vi "FPGA.vi"() -> ()   [LabVIEW 2015]
uses:
  SPI v2/ADXL345 Output.ctl
  <userlib>/_NI SPI IP/FPGA/Controllers/Public/Transfer Settings.ctl
  SPI v2/ADXL345 SPI Statechart.lvsc/Outputs.ctl
  <vilib>/Platform/TimedLoop/XDataNode/timing_clust.ctl
  <vilib>/Platform/TimedLoop/XDataNode/nitl_modes.ctl
  <vilib>/Platform/TimedLoop/XDataNode/wakeup.ctl
  <userlib>/_NI SPI IP/FPGA/Controllers/Public/Spi Master Inputs.ctl
  SPI v2/ADXL345 SPI Statechart.lvsc/Inputs.ctl
  <vilib>/rvi/Emulation/niFpgaGetClockAttributes.vi
  <vilib>/rvi/Emulation/niFpgaSctlEmulationGetInTimedLoop.vi
  <vilib>/rvi/Emulation/niFpgaEmulationReportErrorSimple.vi
  <vilib>/rvi/eio/common/nirviEmuTemplateMethod_errors.vi
  FPGA Globals.vi
  <vilib>/rvi/Emulation/niFpgaCriticalErrorInLSC.vi
  <vilib>/rvi/Emulation/niFpgaProcessEmulError.vi
  SPI v2/ADXL345 SPI Statechart.lvsc/CompanionDiagram.vi/7/SC Main.vi
  <vilib>/eio/EIONode/EIONode.xnode
  <vilib>/rvi/Analysis/measure/butterworth/XNode/niFpgaButterworthFilter.xnode
  <vilib>/Platform/TimedLoop/XDataNode/XDataNode.xnode
  SPI v2/ADXL345 SPI Statechart.lvsc/Trigger.ctl
  <vilib>/Statechart/Infrastructure/RTStatechart/RunTime SCN.xnode
  SPI v2/ADXL345 SPI Statechart.lvsc
  <vilib>/Platform/TimedLoop/XDataNode/XDNodeRunTimeDep.lvlib
  <userlib>/_NI SPI IP/FPGA/Controllers/NI SPI IP FPGA.lvlib
panel:
  out "PWM Out OFF":bool=TRUE
  out "PWM Duty":fxp<+/-,23,14>=336.0
  out "PWM Loop Clock":fxp<+,16,16>
  out "PWM Out ON":bool=TRUE
  in  "BMSTemp":fxp<+,16,8>
  in  "bSBRIOOK3":bool
  in  "bPO2":bool
  in  "bPO3":bool
  out "VHighCurrent":fxp<+/-,36,9>
  out "VLowCurrent":fxp<+/-,36,9>
  in  "bDCDCDisable":bool
  in  "bLapBeaconPickupEnable":bool
  in  "bWheelSpeedsEnable":bool
  out "bLapBeaconPickup":bool
  out "tLapDelta":u32
  in  "bResetFastestLap":bool
  out "tFastestLap":u32
  in  "tLapReference":u32
  in  "bWheelFRFail":bool
  in  "bWheelFLFail":bool
  out "ADXL345 Output":T1
  out "rSlipFR":fxp<+/-,12,1>
  out "rSlipFL":fxp<+/-,12,1>
  out "rSlipRR":fxp<+/-,12,1>
  out "rSlipRL":fxp<+/-,12,1>
  out "sLap":fxp<+,32,12>
  out "vCar":fxp<+/-,33,19>
  out "vAxleF":fxp<+/-,33,19>
  in  "bAccel":bool
  out "vWheelHighest":fxp<+/-,32,18>
  out "vWheelLowest":fxp<+/-,32,18>
  out "vWheelFL":fxp<+/-,32,18>
  out "vWheelFR":fxp<+/-,32,18>
  out "vWheelRL":fxp<+/-,32,18>
  out "vWheelRR":fxp<+/-,32,18>
  in  "Tire Diameter(m)":fxp<+,16,1>
  out "nWheelRR":fxp<+/-,29,16>
  out "nWheelRL":fxp<+/-,29,16>
  out "nWheelFR":fxp<+/-,29,16>
  out "nWheelFL":fxp<+/-,29,16>
  out "NLap":u8
  in  "bResetNLap":bool
  out "aSteerWheel":fxp<+/-,22,10>=124.904541015625
  in  "VSteerWheelMiddle":fxp<+/-,26,5>=0.34827280044555664
  out "bBrakeFOK":bool
  out "bBrakeROK":bool
  out "bLowCurrentOK":bool
  out "bHighCurrentOK":bool
  out "pBrakeF":fxp<+,26,13>
  out "pBrakeR":fxp<+,26,13>
  out "ILowCurrent":fxp<+/-,19,15>=4.375
  out "IHighCurrent":fxp<+/-,19,15>=-20.75
  out "VShockFL":fxp<+/-,24,5>=0.3892974853515625
  out "VShockFR":fxp<+/-,24,5>=0.3425788879394531
  out "VShockRL":fxp<+/-,24,5>=0.3444976806640625
  out "VShockRR":fxp<+/-,24,5>=0.3793773651123047
  in  "bBrakeLight":bool=TRUE
  out "tWheelFLPeriod":u32
  out "tWheelFRPeriod":u32
  out "tWheelRRPeriod":u32
  out "tWheelRLPeriod":u32
  out "bWheelFLStopped":bool=TRUE
  out "bWheelFRStopped":bool=TRUE
  out "bWheelRLStopped":bool=TRUE
  out "bWheelRRStopped":bool=TRUE
  out "VBrakePressureF":fxp<+/-,24,5>=0.4808177947998047
  out "VBrakePressureR":fxp<+/-,24,5>=0.4820976257324219
  out "bWheelFL":bool
  out "bWheelFR":bool
  out "bWheelRR":bool
  out "bWheelRL":bool
  out "V5VSupply":fxp<+/-,24,5>
  in  "tLapMin":u32=15000
  out "tLastLap":u32
  out "bNewLap":bool
  out "tCurrentLap":u32
  in  "bMotorControllerEnable":bool
  out "bTSMSOutStatus":bool
  in  "bSBRIOOK1":bool
  in  "bSBRIOOK2":bool
  out "bBSPDOK":bool
  out "bIMDOK":bool
  out "bBMSOK":bool
  in  "bPosAIREnable":bool
  out "bTSMSInStatus":bool
  in  "bRTDSEnable":bool
  in  "bCoolantPumpEnable":bool
  in  "rTPS1Min":fxp<+,16,4>=0.39990234375
  in  "rTPS1Max":fxp<+,16,4>=0.6201171875
  in  "rTPS2Min":fxp<+,16,4>=0.489990234375
  in  "rTPS2Max":fxp<+,16,4>=0.27001953125
  out "rTPS1":fxp<+/-,31,22>
  out "VTPS1":fxp<+/-,36,9>=3.619058609008789
  out "rTPS2":fxp<+/-,31,22>
  out "VTPS2":fxp<+/-,36,9>=1.0001773834228516
  out "rThrottle":fxp<+/-,33,22>
  out "bTPSInRange":bool
  out "bTPSConsistent":bool
  out "rTPS1Unscaled":fxp<+/-,16,1>
  out "rTPS2Unscaled":fxp<+/-,16,1>
  out "TSBRIO":fxp<+,19,8>=27.25 format="%.10g"
  out "bFPGALED":bool
  out "VsbRIOSupply":fxp<+/-,25,6>=13.101043701171875
  in  "VSupplyOffset":fxp<+,12,4>=8.890625
  in  "stop":bool
  out "Tick Count(mSec)":u32
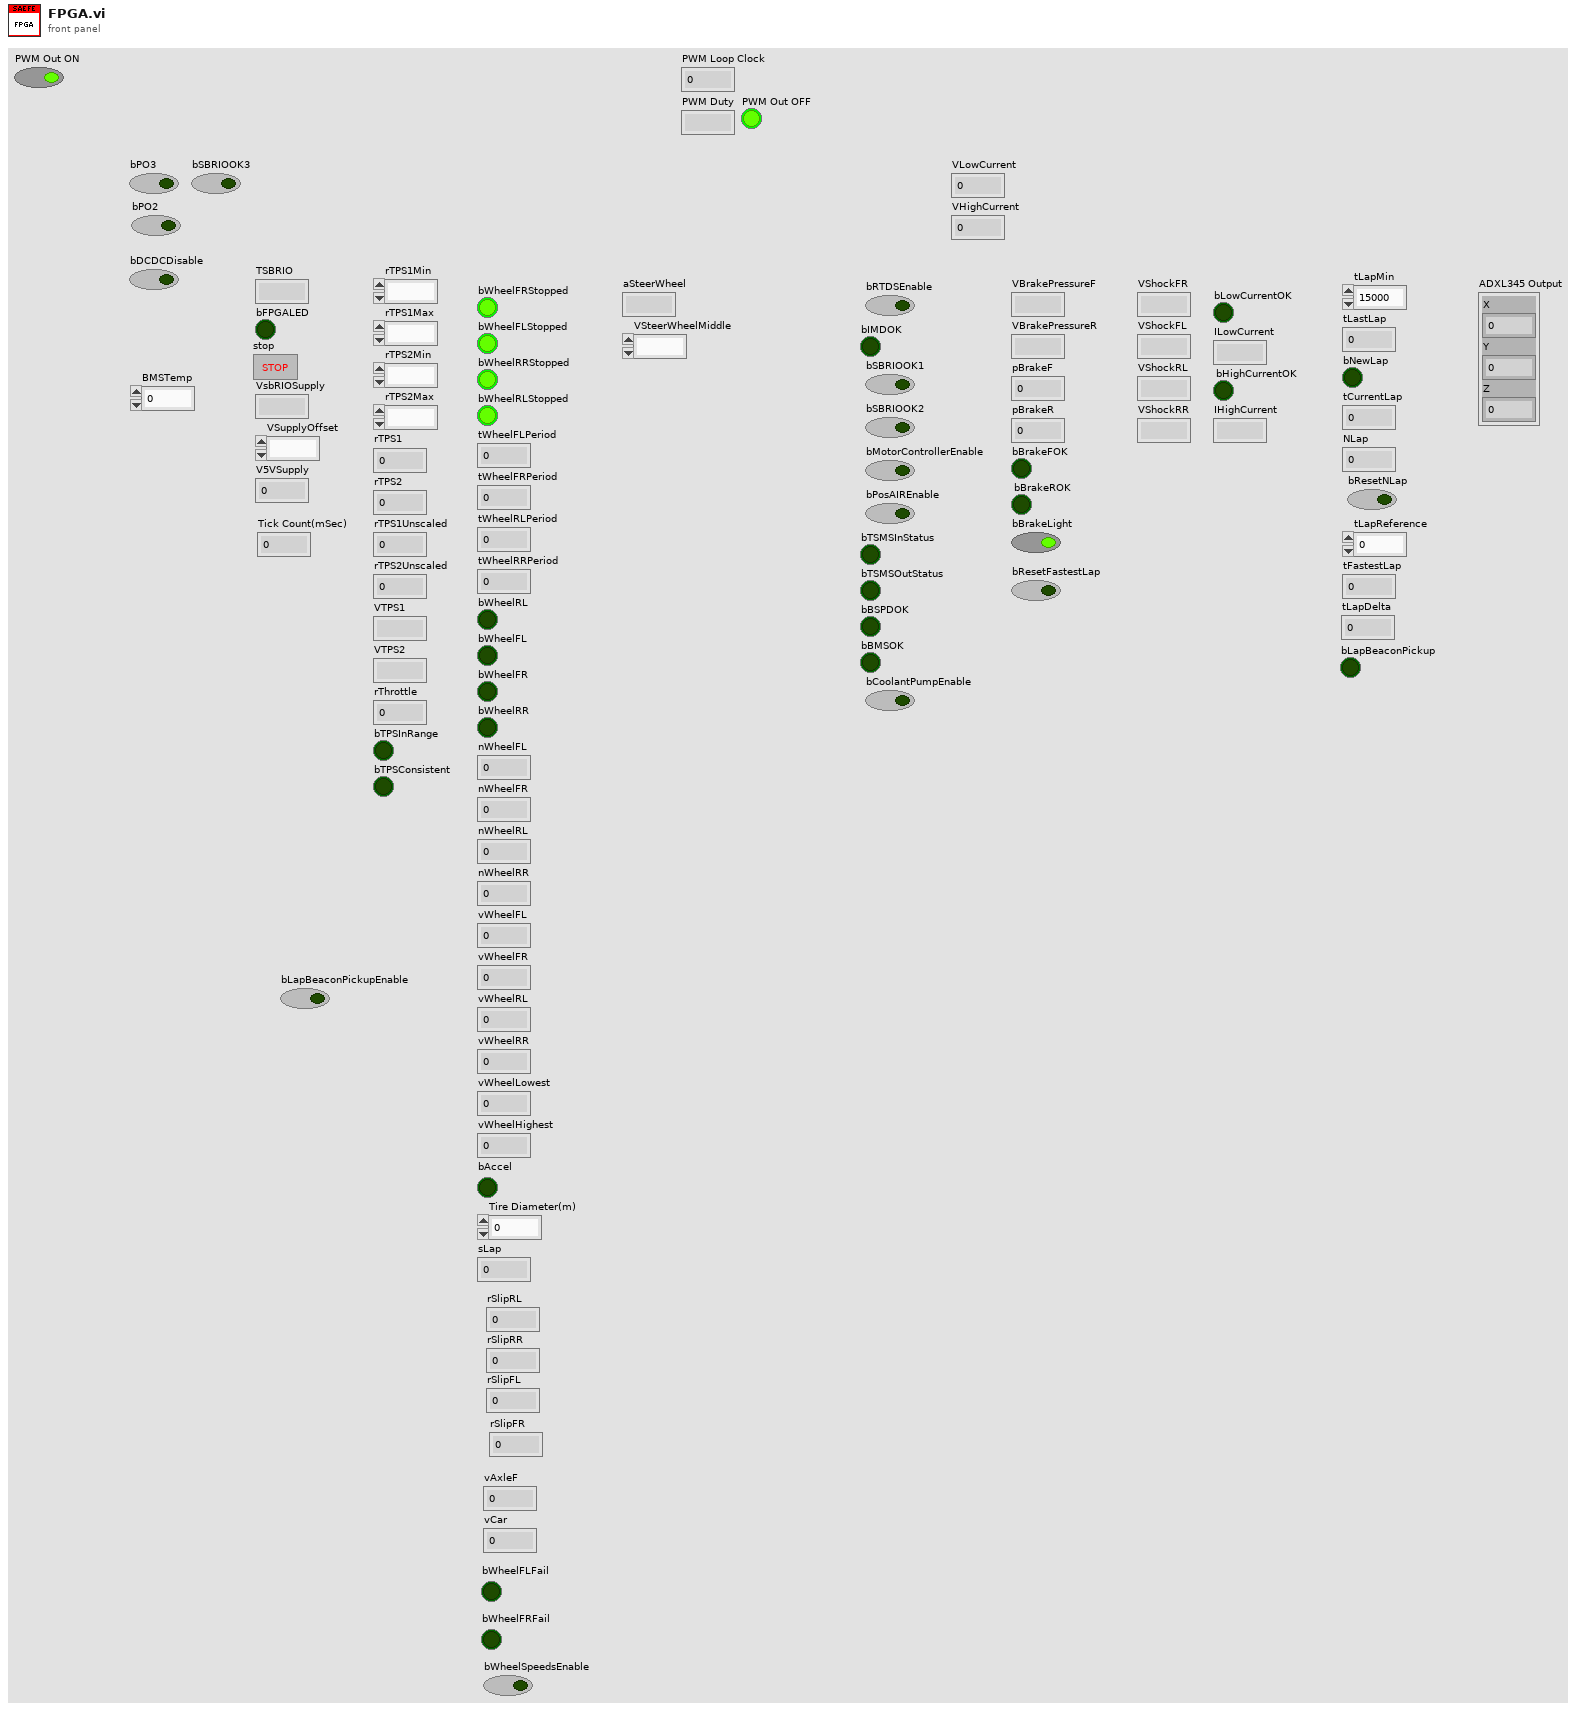
[diagram p1: front panel]
types:
  T1 = typedef "ADXL345 Output.ctl" = cluster{"X":fxp<+/-,14,4>, "Y":fxp<+/-,14,4>, "Z":fxp<+/-,14,4>}
  T2 = typedef "ADXL345 SPI Statechart.lvsc/Outputs.ctl" = cluster{"Transfer Length (bits)":u8, "start strobe":bool, "data to write":u64, "ADXL345 Output":T1}
  T3 = typedef "NI SPI IP FPGA.lvlib/Transfer Settings.ctl" = cluster{"Divide Value":u8, "Transfer Length (bits)":u8, "CS Asserted Polarity":bool, "Clock Polarity (CPOL)":bool, "Clock Phase (CPHA)":bool, "Lengthen MISO Setup":bool, "Direction Change Bit":u8, "MOSI Starts as Output":bool, "Tristatable MOSI":bool}
  T4 = typedef "ADXL345 SPI Statechart.lvsc/Inputs.ctl" = cluster{"read data valid":bool, "read data":u64, "ready for input":bool}
  T5 = typedef "NI SPI IP FPGA.lvlib/Spi Master Inputs.ctl" = cluster{"MISO":bool}
  T6 = typedef "XDNodeRunTimeDep.lvlib/timing_clust.ctl" = cluster{"Expected End [f-1]":u64, "Actual End [f-1]":u64, "Finished Late? [f-1]":bool, "Expected End [i-1]":u64, "Actual End [i-1]":u64, "Finished Late? [i-1]":bool, "Expected Start [i]":u64, "Actual Start [i]":u64, "Expected Start [f]":u64, "Actual Start [f]":u64, "Source Name":string, "Structure Name":string, "Period":i64, "Deadline":i64, "Offset":i64, "Start":i64, "Priority":i32, "Timeout":i32, "Mode":T7, "Wakeup Reason":T8, "Error":errorcluster, "Source Type":string, "Secondary Source Type":string, "Global End Time":u64, "Global Start Time":u64, "Frame Duration":u64, "Iteration Duration":u64, "Assigned CPU":i32, "I/O Scan Engine Mode":u32}
  T7 = typedef "XDNodeRunTimeDep.lvlib/nitl_modes.ctl" = enum32{"No Change", "Process missed periods, maintain original phase", "Discard missed periods, maintain original phase", "Process missed periods, ignore original phase", "Discard missed periods, ignore original phase"}
  T8 = typedef "XDNodeRunTimeDep.lvlib/wakeup.ctl" = enum32{"Normal", "Aborted", "Asynchronous wakeup", "Timing source error", "Timed loop error", "Timeout"}
  T9 = typedef "NI SPI IP FPGA.lvlib/Spi Master Outputs.ctl" = cluster{"Chip Select":bool, "Clock":bool, "MOSI":bool, "MOSI OE":bool}
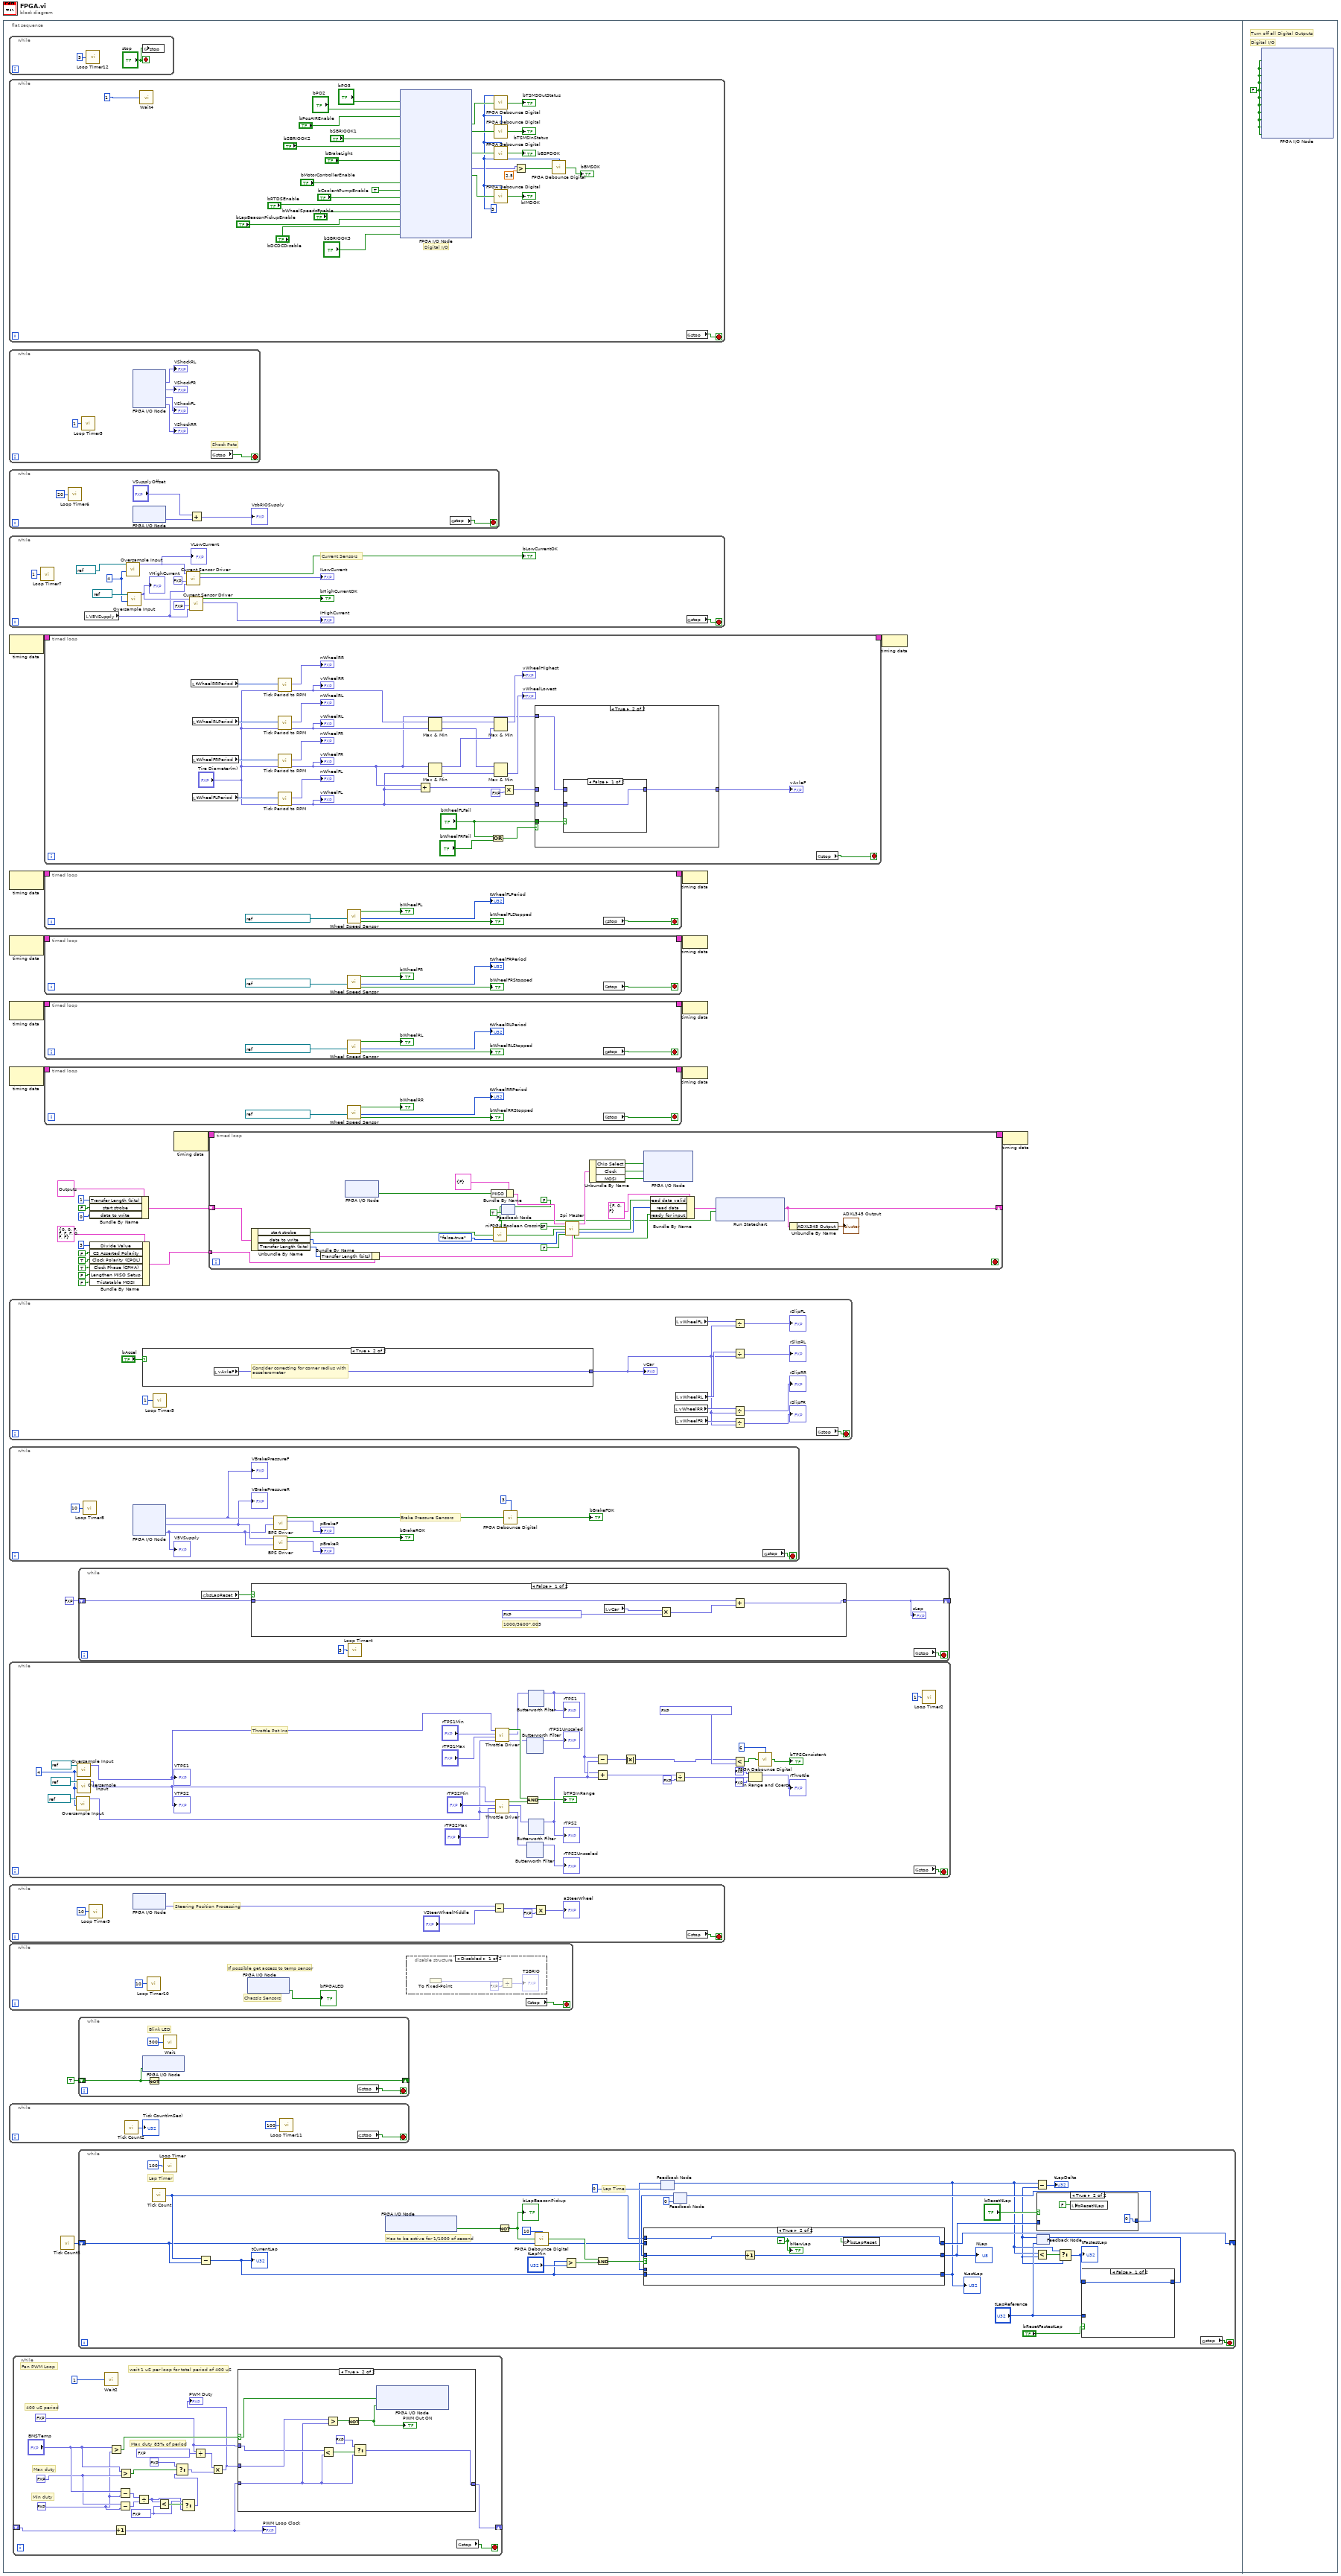
[diagram p0: block diagram]
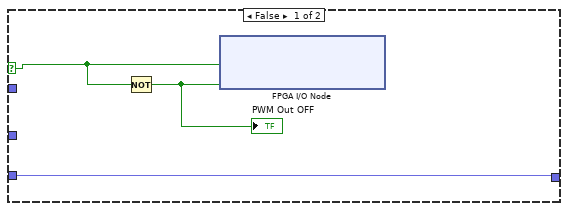
[diagram p2: hidden frame]
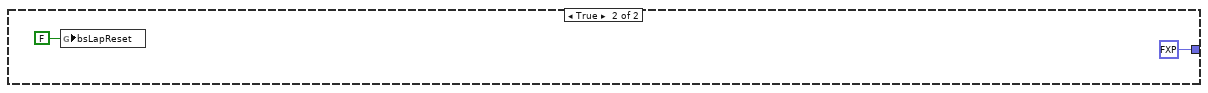
[diagram p3: hidden frame]
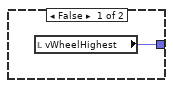
[diagram p4: hidden frame]
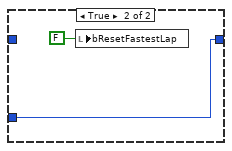
[diagram p7: hidden frame]
diagram:
  n1 = flat-sequence {
    frame #0 {
      n2 = while {
        stop <- "stop" stop-if-true
        n3 = call "Loop Timer12"("Count(mSec)"=u32 5) -> ()  [unwired: 1 out]
        n4 = global write "FPGA Globals.vi" "stop"("stop") -> ()
      }
      n5 = while {
        stop <- w387 stop-if-true
        w364 = u16 3 ("Cycles to Filter")
        # "Digital I/O"
        n6 = call "Wait4"("Count(mSec)"=u32 1) -> ()  [unwired: 1 out]
        n7 = xnode "FPGA I/O Node"("RMC Connector/DIO40"="bPO3", "RMC Connector/DIO42"="bPO2", "RMC Connector/DIO8"="bPosAIREnable", "RMC Connector/DIO5"="bSBRIOOK1", "RMC Connector/DIO6"="bSBRIOOK2", "RMC Connector/DIO11"="bBrakeLight", "RMC Connector/DIO33"="bMotorControllerEnable", "RMC Connector/DIO14"=TRUE, "RMC Connector/DIO41"="bCoolantPumpEnable", "RMC Connector/DIO43"="bRTDSEnable", "RMC Connector/DIO83"="bWheelSpeedsEnable", "RMC Connector/DIO4"="bLapBeaconPickupEnable", "RMC Connector/DIO45"="bDCDCDisable", "RMC Connector/DIO37"="bSBRIOOK3") -> ("RMC Connector/DIO7"=w385:bool, "RMC Connector/DIO39"=w383:bool, "RMC Connector/DIO1"=w372:bool, "AI8"=w362:fxp<+/-,24,5>, "RMC Connector/DIO95"=w379:bool)  [unwired: 19 in, 19 out]
        n8 = call "FPGA Debounce Digital.vi"("Input Signal"=w385, "Cycles to Filter"=w364) -> ("Output Filtered Signal"=→"bTSMSOutStatus":bool)
        n9 = call "FPGA Debounce Digital.vi"("Input Signal"=w383, "Cycles to Filter"=w364) -> ("Output Filtered Signal"=→"bTSMSInStatus":bool)
        n10 = call "FPGA Debounce Digital.vi"("Input Signal"=w372, "Cycles to Filter"=w364) -> ("Output Filtered Signal"=→"bBSPDOK":bool)
        n11 = call "FPGA Debounce Digital.vi"("Input Signal"=w379, "Cycles to Filter"=w364) -> ("Output Filtered Signal"=→"bIMDOK":bool)
        n12 = Greater?(x=w362, y=sgl 2.5) -> (0:w361:bool)
        n13 = call "FPGA Debounce Digital.vi"("Input Signal"=w361, "Cycles to Filter"=w364) -> ("Output Filtered Signal"=→"bBMSOK":bool)
        n14 = global read "FPGA Globals.vi" "stop"() -> (w387:bool)
      }
      n15 = while {
        stop <- w262 stop-if-true
        # "Shock Pots"
        n16 = call "Loop Timer5"("Count(mSec)"=u32 1) -> ()  [unwired: 1 out]
        n17 = xnode "FPGA I/O Node"() -> ("AI9"=→"VShockRL":fxp<+/-,24,5>, "AI10"=→"VShockFR":fxp<+/-,24,5>, "AI11"=→"VShockFL":fxp<+/-,24,5>, "AI8"=→"VShockRR":fxp<+/-,24,5>)  [unwired: 4 in, 4 out]
        n18 = global read "FPGA Globals.vi" "stop"() -> (w262:bool)
      }
      n19 = while {
        stop <- w247 stop-if-true
        n20 = call "Loop Timer6"("Count(mSec)"=u32 20) -> ()  [unwired: 1 out]
        n21 = xnode "FPGA I/O Node"() -> ("AI0"=w250:fxp<+/-,24,5>)  [unwired: 1 in, 1 out]
        n22 = Add(x="VSupplyOffset", y=w250) -> (x+y=→"VsbRIOSupply":fxp<+/-,25,6>)
        n23 = global read "FPGA Globals.vi" "stop"() -> (w247:bool)
      }
      n24 = while {
        stop <- w274 stop-if-true
        w271 = u8 4 ("NSamples")
        # "Current Sensors"
        n25 = call "Loop Timer7"("Count(mSec)"=u32 1) -> ()  [unwired: 1 out]
        n26 = local read "V5VSupply"() -> (w269:fxp<+/-,24,5>)
        n27 = call "Oversample Input.vi"("NSamples"=w271, "Channel"=refnum<k21> "AI2" ("FPGA I/O In")) -> ("Output"=w267:fxp<+/-,36,9>)  [unwired: 9 in]
        "VLowCurrent" <- w267
        n28 = call "Oversample Input.vi"("NSamples"=w271, "Channel"=refnum<k21> "AI1") -> ("Output"=w270:fxp<+/-,36,9>)  [unwired: 9 in]
        "VHighCurrent" <- w270
        n29 = call "Current Sensor Driver.vi"("VSupply"=w269, "IRange"=fxp<+,27,10> 50.0 ("Range"), "VInput"=w267) -> ("ISensor"=→"ILowCurrent":fxp<+/-,19,15>, "bSensorOK"=→"bLowCurrentOK":bool)  [unwired: 7 in]
        n30 = call "Current Sensor Driver.vi"("VSupply"=w269, "IRange"=fxp<+,27,10> 600.0 ("Range"), "VInput"=w270) -> ("ISensor"=→"IHighCurrent":fxp<+/-,19,15>, "bSensorOK"=→"bHighCurrentOK":bool)  [unwired: 7 in]
        n31 = global read "FPGA Globals.vi" "stop"() -> (w274:bool)
      }
      n32 = node-c288() -> (w18:T6)  [unwired: 1 in]
      n33 = node-c288() -> (w27:T6)  [unwired: 1 in]
      n34 = node-c288() -> (w25:T6)  [unwired: 1 in]
      n35 = node-c288() -> (w23:T6)  [unwired: 1 in]
      n36 = node-c288() -> (w21:T6)  [unwired: 1 in]
      n37 = while {
        stop <- w122 stop-if-true
        n38 = case shown="True" "bAccel" {
          tunnel: [w123 w124] -> w112
          frame False {
            n39 = local read "vWheelHighest"() -> (w123:fxp<+/-,32,18>)
          }
          frame True {
            # "Consider correcting for corner radius with\naccelerometer"
            n40 = local read "vAxleF"() -> (w124:fxp<+/-,33,19>)
          }
        }
        "vCar" <- w112
        n41 = call "Loop Timer3"("Count(mSec)"=u32 1) -> ()  [unwired: 1 out]
        n42 = local read "vWheelRR"() -> (w117:fxp<+/-,32,18>)
        n43 = local read "vWheelFL"() -> (w115:fxp<+/-,32,18>)
        n44 = local read "vWheelRL"() -> (w119:fxp<+/-,32,18>)
        n45 = local read "vWheelFR"() -> (w113:fxp<+/-,32,18>)
        n46 = Divide(x=w115, y=w112) -> (x/y=→"rSlipFL":fxp<+/-,12,1>)
        n47 = Divide(x=w119, y=w112) -> (x/y=→"rSlipRL":fxp<+/-,12,1>)
        n48 = Divide(x=w117, y=w112) -> (x/y=→"rSlipRR":fxp<+/-,12,1>)
        n49 = Divide(x=w113, y=w112) -> (x/y=→"rSlipFR":fxp<+/-,12,1>)
        n50 = global read "FPGA Globals.vi" "stop"() -> (w122:bool)
      }
      n51 = while {
        stop <- w286 stop-if-true
        # "Brake Pressure Sensors"
        n52 = call "Loop Timer8"("Count(mSec)"=u32 10) -> ()  [unwired: 1 out]
        n53 = xnode "FPGA I/O Node"() -> ("AI3"=w291:fxp<+/-,24,5>, "AI4"=w289:fxp<+/-,24,5>, "AI12"=w284:fxp<+/-,24,5>)  [unwired: 3 in, 3 out]
        "VBrakePressureF" <- w291
        "VBrakePressureR" <- w289
        "V5VSupply" <- w284
        n54 = call "BPS Driver.vi"("Supply Voltage"=w284, "Signal In"=w291) -> ("Brake Pressure (psi)"=→"pBrakeF":fxp<+,26,13>, "Sensor OK?"=w283:bool)  [unwired: 8 in]
        n55 = call "BPS Driver.vi"("Supply Voltage"=w284, "Signal In"=w289) -> ("Brake Pressure (psi)"=→"pBrakeR":fxp<+,26,13>, "Sensor OK?"=→"bBrakeROK":bool)  [unwired: 8 in]
        n56 = call "FPGA Debounce Digital.vi"("Input Signal"=w283, "Cycles to Filter"=u16 3) -> ("Output Filtered Signal"=→"bBrakeFOK":bool)
        n57 = global read "FPGA Globals.vi" "stop"() -> (w286:bool)
      }
      n58 = while {
        stop <- w318 stop-if-true
        w300 = u8 4 ("NSamples")
        # "Throttle Pot Ins"
        n59 = call "Oversample Input.vi"("NSamples"=w300, "Channel"=refnum<k21> "AI12") -> ("Output"=w298:fxp<+/-,36,9>)  [unwired: 9 in]
        n60 = call "Oversample Input.vi"("NSamples"=w300, "Channel"=refnum<k21> "AI6") -> ("Output"=w299:fxp<+/-,36,9>)  [unwired: 9 in]
        "VTPS2" <- w299
        n61 = call "Oversample Input.vi"("NSamples"=w300, "Channel"=refnum<k21> "AI5") -> ("Output"=w296:fxp<+/-,36,9>)  [unwired: 9 in]
        "VTPS1" <- w296
        n62 = call "Throttle Driver.vi"("Reference Voltage In"=w298, "Throttle Max"="rTPS1Max", "Throttle Min"="rTPS1Min", "Throttle Voltage In"=w296) -> ("Unscaled Throttle Percent"=w313:fxp<+/-,16,1>, "Throttle Percent"=w306:fxp<+/-,27,18>, "In Range"=w322:bool)  [unwired: 5 in]
        n63 = call "Throttle Driver.vi"("Reference Voltage In"=w298, "Throttle Max"="rTPS2Max", "Throttle Min"="rTPS2Min", "Throttle Voltage In"=w299) -> ("Unscaled Throttle Percent"=w311:fxp<+/-,16,1>, "Throttle Percent"=w309:fxp<+/-,27,18>, "In Range"=w321:bool)  [unwired: 5 in]
        n64 = xnode "Butterworth Filter"("input data"=w313) -> ("output data"=→"rTPS1Unscaled":fxp<+/-,16,1>)  [unwired: 2 in]
        n65 = xnode "Butterworth Filter"("input data"=w311) -> ("output data"=→"rTPS2Unscaled":fxp<+/-,16,1>)  [unwired: 2 in]
        n66 = Compound Arithmetic op=AND(w322, w321) -> (→"bTPSInRange":bool)
        n67 = xnode "Butterworth Filter"("input data"=w306) -> ("output data"=w305:fxp<+/-,31,22>)  [unwired: 2 in]
        "rTPS1" <- w305
        n68 = xnode "Butterworth Filter"("input data"=w309) -> ("output data"=w308:fxp<+/-,31,22>)  [unwired: 2 in]
        "rTPS2" <- w308
        n69 = Subtract(x=w305, y=w308) -> (x-y=w317:fxp<+/-,32,23>)
        n70 = Add(x=w305, y=w308) -> (x+y=w324:fxp<+/-,32,23>)
        n71 = Absolute Value(x=w317) -> (abs(x)=w293:fxp<+,31,22>)
        n72 = Divide(x=w324, y=fxp<+,1,2> 2.0) -> (x/y=w307:fxp<+/-,33,22>)
        n73 = Less?(x=w293, y=fxp<+/-,46,20> 0.09999999403953552) -> (x < y?=w295:bool)
        n74 = In Range and Coerce(upper limit=fxp<+/-,33,22> 1.0, x=w307, lower limit=fxp<+/-,33,22> 0.0) -> (coerced(x)=→"rThrottle":fxp<+/-,33,22>)  [unwired: 1 out]
        n75 = call "FPGA Debounce Digital.vi"("Input Signal"=w295, "Cycles to Filter"=i16 6) -> ("Output Filtered Signal"=→"bTPSConsistent":bool)
        n76 = global read "FPGA Globals.vi" "stop"() -> (w318:bool)
        n77 = call "Loop Timer2"("Count(mSec)"=u32 1) -> ()  [unwired: 1 out]
      }
      n78 = while {
        stop <- w390 stop-if-true
        # "Steering Position Processing"
        n79 = call "Loop Timer9"("Count(mSec)"=u32 10) -> ()  [unwired: 1 out]
        n80 = xnode "FPGA I/O Node"() -> ("AI14"=w395:fxp<+/-,24,5>)  [unwired: 1 in, 1 out]
        n81 = Subtract(x=w395, y="VSteerWheelMiddle") -> (x-y=w393:fxp<+/-,27,6>)
        n82 = Multiply(x=w393, y=fxp<+,4,7> 72.0) -> (x*y=→"aSteerWheel":fxp<+/-,22,10>)
        n83 = global read "FPGA Globals.vi" "stop"() -> (w390:bool)
      }
      n84 = while {
        stop <- w257 stop-if-true
        # "If possible get access to temp sensor"
        # "Chassis Sensors"
        n85 = call "Loop Timer10"("Count(mSec)"=u32 10) -> ()  [unwired: 1 out]
        n86 = xnode "FPGA I/O Node"() -> ("FPGA LED"=→"bFPGALED":bool)  [unwired: 1 in, 1 out]
        n87 = disable-structure shown="Disabled" {
          frame Disabled {
            n88 = To Fixed-Point() -> (fixed-point=w259:fxp<+/-,16,9>)  [unwired: 2 in]
            n89 = Divide(x=w259, y=fxp<+/-,16,9> 4.0) -> (x/y=→"TSBRIO":fxp<+,19,8>)
          }
          frame Enabled {
          }
        }
        n90 = global read "FPGA Globals.vi" "stop"() -> (w257:bool)
      }
      n91 = while {
        stop <- w242 stop-if-true
        n92 = call "Tick Count2"() -> ("Tick Count(mSec)"=→"Tick Count(mSec)":u32)
        n93 = call "Loop Timer11"("Count(uSec)"=u32 100) -> ()  [unwired: 1 out]
        n94 = global read "FPGA Globals.vi" "stop"() -> (w242:bool)
      }
      n95 = while {
        shift-right: [w41] -> _
        shift-left: _ -> [w42]
        stop <- w40 stop-if-true
        w31 = fxp<+,5,-1> 0.40625
        w38 = fxp<+,5,9> 400.0
        w47 = fxp<+,3,6> 40.0 ("Temp 2")
        w48 = fxp<+,6,6> 55.0 ("Temp 2")
        # "400 uS period"
        # "wait 1 uS per loop for total period of 400 uS"
        # "Max duty 85% of period"
        # "Fan PWM Loop"
        # "Min duty"
        # "Max duty"
        n96 = call "Wait2"("Count(uSec)"=u8 1) -> ()  [unwired: 1 out]
        n97 = Greater?(x="BMSTemp", y=w47) -> (0:w43:bool)
        n98 = Increment(x=w42) -> (x+1=w36:fxp<+,16,16>)
        "PWM Loop Clock" <- w36
        n99 = Subtract(x="BMSTemp", y=w47) -> (x-y=w34:fxp<+/-,17,9>)
        n100 = Subtract(x=w48, y=w47) -> (x-y=w33:fxp<+,4,4>)
        n101 = Greater?(x="BMSTemp", y=w48) -> (0:w50:bool)
        n102 = Divide(x=w34, y=w33) -> (x/y=w30:fxp<+/-,17,5>)
        n103 = Less?(x=w30, y=w31) -> (x < y?=w32:bool)
        n104 = Select(t=w31, s=w32, f=w30) -> (s? t:f=w29:fxp<+/-,17,5>)
        n105 = Select(t=fxp<+,1,1> 1.0, s=w50, f=w29) -> (s? t:f=w46:fxp<+/-,17,5>)
        n106 = Divide(x=w38, y=fxp<+,19,1> 1.1764717102050781 ("Temp 2")) -> (x/y=w44:fxp<+,6,9>)
        n107 = Multiply(x=w44, y=w46) -> (x*y=w35:fxp<+/-,23,14>)
        "PWM Duty" <- w35
        n108 = case shown="True" w43 {
          selector: w43 -> [w52 w62]
          tunnel: w35 -> [_ w61]
          tunnel: w36 -> [w53 w56]
          tunnel: [w53 w58] -> w41
          tunnel: w38 -> [_ w57]
          frame False {
            n109 = Not(x=w52) -> (.not. x?=w51:bool)
            "PWM Out OFF" <- w51
            n110 = xnode "FPGA I/O Node"("RMC Connector/DIO9"=w52, "RMC Connector/DIO10"=w51) -> ()  [unwired: 2 in, 2 out]
          }
          frame True {
            n111 = Less?(x=w57, y=w56) -> (x < y?=w59:bool)
            n112 = Greater?(x=w61, y=w56) -> (0:w55:bool)
            n113 = Not(x=w55) -> (.not. x?=w54:bool)
            "PWM Out ON" <- w54
            n114 = Select(t=fxp<+,1,1> 0.0, s=w59, f=w56) -> (s? t:f=w58:fxp<+,16,16>)
            n115 = xnode "FPGA I/O Node"("RMC Connector/DIO9"=w62, "RMC Connector/DIO10"=w54) -> ()  [unwired: 2 in, 2 out]
          }
        }
        n116 = global read "FPGA Globals.vi" "stop"() -> (w40:bool)
      }
      n117 = timed-loop {
        timing: w18 -> [_]
        timing-out: [_] -> w17
        stop <- w145 stop-if-true
        n118 = local read "tWheelRRPeriod"() -> (w146:u32)
        n119 = local read "tWheelRLPeriod"() -> (w147:u32)
        n120 = local read "tWheelFRPeriod"() -> (w148:u32)
        n121 = local read "tWheelFLPeriod"() -> (w149:u32)
        n122 = call "Tick Period to RPM.vi"("Tire Diameter(m)"="Tire Diameter(m)", "Tick Period"=w146) -> ("vWheel"=w142:fxp<+/-,32,18>, "nWheel"=→"nWheelRR":fxp<+/-,29,16>)  [unwired: 8 in]
        "vWheelRR" <- w142
        n123 = call "Tick Period to RPM.vi"("Tire Diameter(m)"="Tire Diameter(m)", "Tick Period"=w147) -> ("vWheel"=w141:fxp<+/-,32,18>, "nWheel"=→"nWheelRL":fxp<+/-,29,16>)  [unwired: 8 in]
        "vWheelRL" <- w141
        n124 = call "Tick Period to RPM.vi"("Tire Diameter(m)"="Tire Diameter(m)", "Tick Period"=w148) -> ("vWheel"=w128:fxp<+/-,32,18>, "nWheel"=→"nWheelFR":fxp<+/-,29,16>)  [unwired: 8 in]
        "vWheelFR" <- w128
        n125 = call "Tick Period to RPM.vi"("Tire Diameter(m)"="Tire Diameter(m)", "Tick Period"=w149) -> ("vWheel"=w127:fxp<+/-,32,18>, "nWheel"=→"nWheelFL":fxp<+/-,29,16>)  [unwired: 8 in]
        "vWheelFL" <- w127
        n126 = Add(x=w128, y=w127) -> (x+y=w134:fxp<+/-,33,19>)
        n127 = Max & Min(x=w142, y=w141) -> (max(x,y)=w139:fxp<+/-,32,18>, min(x,y)=w138:fxp<+/-,32,18>)
        n128 = Max & Min(x=w128, y=w127) -> (max(x,y)=w140:fxp<+/-,32,18>, min(x,y)=w137:fxp<+/-,32,18>)
        n129 = Or(x="bWheelFLFail", y="bWheelFRFail") -> (x .or. y?=w126:bool)
        n130 = Max & Min(x=w139, y=w140) -> (max(x,y)=→"vWheelHighest":fxp<+/-,32,18>)  [unwired: 1 out]
        n131 = Max & Min(x=w138, y=w137) -> (min(x,y)=→"vWheelLowest":fxp<+/-,32,18>)  [unwired: 1 out]
        n132 = Multiply(x=w134, y=fxp<+/-,33,19> 0.5) -> (x*y=w131:fxp<+/-,33,19>)
        n133 = case shown="True" w126 {
          tunnel: w131 -> [w152 _]
          tunnel: [w152 w154] -> w130
          tunnel: "bWheelFLFail" -> [_ w156]
          tunnel: w128 -> [_ w155]
          tunnel: w127 -> [_ w153]
          frame False {
          }
          frame True {
            n134 = case shown="False" w156 {
              tunnel: w155 -> [_ w158]
              tunnel: [w157 w158] -> w154
              tunnel: w153 -> [w157 _]
              frame False {
              }
              frame True {
              }
            }
          }
        }
        "vAxleF" <- w130
        n135 = global read "FPGA Globals.vi" "stop"() -> (w145:bool)
      }
      n136 = timed-loop {
        timing: w27 -> [_]
        timing-out: [_] -> w26
        stop <- w232 stop-if-true
        n137 = call "Wheel Speed Sensor.vi"("FPGA I/O In"=refnum<k21> "RMC Connector/DIO88") -> ("Stopped"=→"bWheelFLStopped":bool, "Tick Period"=→"tWheelFLPeriod":u32, "State Out"=→"bWheelFL":bool)  [unwired: 8 in]
        n138 = global read "FPGA Globals.vi" "stop"() -> (w232:bool)
      }
      n139 = timed-loop {
        timing: w25 -> [_]
        timing-out: [_] -> w24
        stop <- w224 stop-if-true
        n140 = call "Wheel Speed Sensor.vi"("FPGA I/O In"=refnum<k21> "RMC Connector/DIO87") -> ("Stopped"=→"bWheelFRStopped":bool, "Tick Period"=→"tWheelFRPeriod":u32, "State Out"=→"bWheelFR":bool)  [unwired: 8 in]
        n141 = global read "FPGA Globals.vi" "stop"() -> (w224:bool)
      }
      n142 = timed-loop {
        timing: w23 -> [_]
        timing-out: [_] -> w22
        stop <- w215 stop-if-true
        n143 = call "Wheel Speed Sensor.vi"("FPGA I/O In"=refnum<k21> "RMC Connector/DIO86") -> ("Stopped"=→"bWheelRLStopped":bool, "Tick Period"=→"tWheelRLPeriod":u32, "State Out"=→"bWheelRL":bool)  [unwired: 8 in]
        n144 = global read "FPGA Globals.vi" "stop"() -> (w215:bool)
      }
      n145 = timed-loop {
        timing: w21 -> [_]
        timing-out: [_] -> w20
        stop <- w206 stop-if-true
        n146 = call "Wheel Speed Sensor.vi"("FPGA I/O In"=refnum<k21> "RMC Connector/DIO85") -> ("Stopped"=→"bWheelRRStopped":bool, "Tick Period"=→"tWheelRRPeriod":u32, "State Out"=→"bWheelRR":bool)  [unwired: 8 in]
        n147 = global read "FPGA Globals.vi" "stop"() -> (w206:bool)
      }
      n148 = call "Tick Count3"() -> ("Tick Count(mSec)"=w19:u32)
      n149 = while {
        shift-right: [w99] -> _
        shift-left: fxp<+,32,12> 0.0 -> [w100]
        stop <- w103 stop-if-true
        n150 = global read "FPGA Globals.vi" "bsLapReset"() -> (w101:bool)
        n151 = case shown="False" w101 {
          tunnel: w100 -> [w105 _]
          tunnel: [w104 fxp<+,32,12> 0.0] -> w99
          frame False {
            # "1000/3600*.005"
            n152 = local read "vCar"() -> (w108:fxp<+/-,33,19>)
            n153 = Multiply(x=w108, y=fxp<+,32,4> 0.00138888880610466) -> (x*y=w106:fxp<+,32,12>)
            n154 = Add(x=w105, y=w106) -> (x+y=w104:fxp<+,32,12>)
          }
          frame True {
            n155 = global write "FPGA Globals.vi" "bsLapReset"(FALSE ("bsLapReset")) -> ()
          }
        }
        "sLap" <- w99
        n156 = call "Loop Timer4"("Count(mSec)"=u32 5) -> ()  [unwired: 1 out]
        n157 = global read "FPGA Globals.vi" "stop"() -> (w103:bool)
      }
      n158 = while {
        shift-right: [w252] -> _
        shift-left: TRUE ("FPGA LED") -> [w253]
        stop <- w251 stop-if-true
        # "Blink LED"
        n159 = xnode "FPGA I/O Node"("FPGA LED"=w253) -> ()  [unwired: 1 in, 1 out]
        n160 = Not(x=w253) -> (.not. x?=w252:bool)
        n161 = call "Wait"("Count(mSec)"=u32 500) -> ()  [unwired: 1 out]
        n162 = global read "FPGA Globals.vi" "stop"() -> (w251:bool)
      }
      n163 = while {
        shift-right: [w179] -> _
        shift-left: w19 -> [w178]
        stop <- w188 stop-if-true
        # "Lap Time"
        # "Lap Timer"
        # "Has to be active for 1/1000 of second"
        n164 = call "Tick Count"() -> ("Tick Count(mSec)"=w180:u32)
        n165 = call "Loop Timer"("Count(uSec)"=u32 100) -> ()  [unwired: 1 out]
        n166 = Subtract(x=w180, y=w178) -> (x-y=w183:u32)
        "tCurrentLap" <- w183
        n167 = xnode "FPGA I/O Node"() -> ("RMC Connector/DIO12"=w163:bool)  [unwired: 1 in, 1 out]
        n168 = Not(x=w163) -> (.not. x?=w164:bool)
        "bLapBeaconPickup" <- w164
        n169 = call "FPGA Debounce Digital.vi"("Input Signal"=w164, "Cycles to Filter"=u16 10) -> ("Output Filtered Signal"=w186:bool)
        n170 = Greater?(x=w183, y="tLapMin") -> (0:w185:bool)
        n171 = And(x=w186, y=w185) -> (x .and. y?=w184:bool)
        n172 = feedback #1(u32 0) -> (w181:u32)
        n173 = feedback #2(u8 0) -> (w176:u8)
        n174 = case shown="True" w184 {
          tunnel: w183 -> [_ w204]
          tunnel: [w199 w204] -> w167
          tunnel: w181 -> [w199 _]
          tunnel: w180 -> [_ w203]
          tunnel: [w198 w203] -> w179
          tunnel: w178 -> [w198 _]
          tunnel: w176 -> [w197 w202]
          tunnel: [w197 w201] -> w174
          frame False {
          }
          frame True {
            w200 = TRUE
            n175 = Increment(x=w202) -> (x+1=w201:u8)
            n176 = global write "FPGA Globals.vi" "bsLapReset"(w200) -> ()
            "bNewLap" <- w200
          }
        }
        "tLastLap" <- w167
        "NLap" <- w174
        n177 = feedback-in #1(w167) -> ()
        n178 = case shown="True" "bResetNLap" {
          tunnel: w174 -> [w194 _]
          tunnel: [w194 u8 0] -> w173
          frame False {
          }
          frame True {
            n179 = local write "bResetNLap"(FALSE ("bResetNLap")) -> ()
          }
        }
        n180 = feedback-in #2(w173) -> ()
        n181 = feedback #3("tLapReference") -> (w166:u32)
        n182 = Subtract(x=w167, y=w166) -> (x-y=→"tLapDelta":u32)
        n183 = Less?(x=w167, y=w166) -> (x < y?=w172:bool)
        n184 = Select(t=w167, s=w172, f=w166) -> (s? t:f=w170:u32)
        "tFastestLap" <- w170
        n185 = case shown="False" "bResetFastestLap" {
          tunnel: w170 -> [w191 _]
          tunnel: "tLapReference" -> [_ w192]
          tunnel: [w191 w192] -> w168
          frame False {
          }
          frame True {
            n186 = local write "bResetFastestLap"(FALSE ("bResetFastestLap")) -> ()
          }
        }
        n187 = feedback-in #3(w168) -> ()
        n188 = global read "FPGA Globals.vi" "stop"() -> (w188:bool)
      }
      n189 = Bundle By Name(cluster=T2 {"Transfer Length (bits)"=0, "start strobe"=FALSE, "data to write"=0, "ADXL345 Output"={"X"=0.0, "Y"=0.0, "Z"=0.0}} ("Outputs"), "Transfer Length (bits)"=u8 1, "start strobe"=FALSE, "data to write"=u64 0) -> (w4:T2)
      n190 = Bundle By Name(cluster=T3 {"Divide Value"=0, "Transfer Length (bits)"=0, "CS Asserted Polarity"=FALSE, "Clock Polarity (CPOL)"=FALSE, "Clock Phase (CPHA)"=FALSE, "Lengthen MISO Setup"=FALSE, "Direction Change Bit"=0, "MOSI Starts as Output"=FALSE, "Tristatable MOSI"=FALSE} ("spi transfer settings"), "Divide Value"=u8 3, "CS Asserted Polarity"=FALSE, "Clock Polarity (CPOL)"=TRUE, "Clock Phase (CPHA)"=TRUE, "Lengthen MISO Setup"=FALSE, "Tristatable MOSI"=FALSE) -> (w10:T3)
      n191 = node-c288() -> (w15:T6)  [unwired: 1 in]
      n192 = timed-loop {
        timing: w15 -> [_]
        timing-out: [_] -> w14
        tunnel: w10 -> [w73]
        shift-right: [w64] -> _
        shift-left: w4 -> [w75]
        stop <- _ stop-if-true
        n193 = Unbundle By Name(w75) -> ("start strobe"=w69:bool, "data to write"=w70:u64, "Transfer Length (bits)"=w71:u8)
        n194 = Bundle By Name(cluster=w73, "Transfer Length (bits)"=w71) -> (w72:T3)
        n195 = xnode "FPGA I/O Node"() -> ("MISO"=w88:bool)  [unwired: 1 in, 1 out]
        n196 = Bundle By Name(cluster=T5 {"MISO"=FALSE} ("spi input"), "MISO"=w88) -> (w87:T5)
        n197 = feedback-in #4(FALSE) -> ()
        n198 = feedback #4(TRUE) -> (w66:bool)
        n199 = call <vilib>:"niFPGA Boolean Crossing.vi"("input"=w69, "direction"=enum8{"either", "false-true", "true-false"}."false-true", "initialize"=w66) -> ("crossing"=w68:bool)  [unwired: 6 in]
        n200 = call <userlib>:"Spi Master.vi"("spi input"=w87, "manual assert chip select"=FALSE, "start strobe"=w68, "data to write"=w70, "MOSI output enable done"=FALSE, "spi transfer settings"=w72) -> ("spi output"=w79:T9, "read data valid"=w85:bool, "read data"=w84:u64, "ready for input"=w83:bool)  [unwired: 6 in]
        n201 = Unbundle By Name(w79) -> ("Chip Select"=w78:bool, "Clock"=w77:bool, "MOSI"=w76:bool)
        n202 = xnode "FPGA I/O Node"("ACCEL Select"=w78, "CLK"=w77, "MOSI"=w76) -> ()  [unwired: 3 in, 3 out]
        n203 = Bundle By Name(cluster=T4 {"read data valid"=FALSE, "read data"=0, "ready for input"=FALSE} ("Inputs"), "read data valid"=w85, "read data"=w84, "ready for input"=w83) -> (w82:T4)
        n204 = xnode "Run Statechart"("Init?"=w66, "Inputs"=w82) -> ("Outputs"=w64:T2)  [unwired: 1 in, 1 out]
        n205 = Unbundle By Name(w64) -> ("ADXL345 Output"=→"ADXL345 Output":T1)
      }
      n206 = node-c288(w26) -> ()
      n207 = node-c288(w24) -> ()
      n208 = node-c288(w22) -> ()
      n209 = node-c288(w20) -> ()
      n210 = node-c288(w17) -> ()
      n211 = node-c288(w14) -> ()
    }
    frame #1 {
      w396 = FALSE
      # "Turn off all Digital Outputs"
      # "Digital I/O"
      n212 = xnode "FPGA I/O Node"("RMC Connector/DIO8"=w396, "RMC Connector/DIO6"=w396, "RMC Connector/DIO5"=w396, "RMC Connector/DIO40"=w396, "RMC Connector/DIO40"=w396, "RMC Connector/DIO11"=w396, "RMC Connector/DIO33"=w396, "RMC Connector/DIO14"=w396, "RMC Connector/DIO41"=w396, "RMC Connector/DIO11"=w396, "RMC Connector/DIO9"=w396) -> ()  [unwired: 11 in, 11 out]
    }
  }
